vi "GetDisabledInputs.vi"(6 "error in":errorcluster, 9 "IndexArray in":refnum<class "IndexArray.lvclass">) -> (0 "error out":errorcluster, 3 "IndexArray out":refnum<class "IndexArray.lvclass">, 4 "indices":string)   [LabVIEW 2014, in "IndexArray.lvclass"]
uses:
  IndexArray.lvclass
  Python/Parsing/ListTypesTD.ctl
  Python/Parsing/Python Functions.lvlib
  Python/PythonConfiguration/PythonConfiguration.lvclass
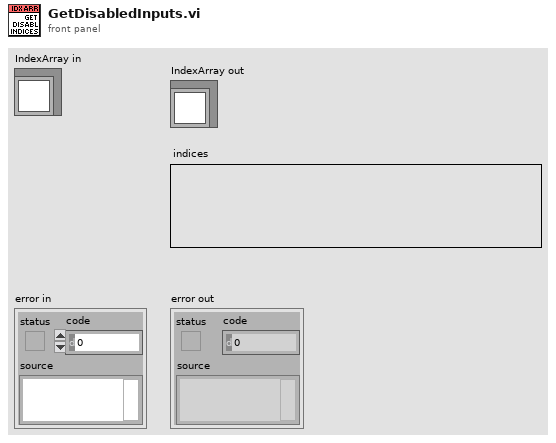
[diagram p1: front panel]
types:
  T1 = typedef "Python Functions.lvlib/ListTypesTD.ctl" = enum16{"list", "tuple", "parameter list", "output list", "return values"}
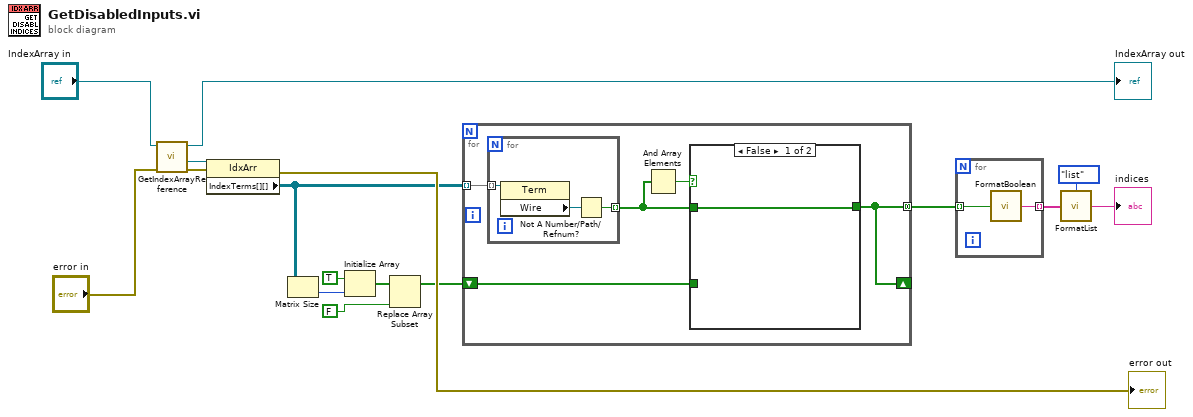
[diagram p0: block diagram]
diagram:
  n1 = call "GetIndexArrayReference.vi"("error in"="error in", "Index Array in"="IndexArray in") -> ("error out"=w13:errorcluster, "reference out"=w14:refnum<vi>, "Index Array out"=→"IndexArray out":refnum<class "IndexArray.lvclass">)  [unwired: 7 in]
  n2 = property class="IdxArr"(reference=w14, error in=w13) -> (error out=→"error out":errorcluster, "IndexTerms[][]"=w2:refnum<vi>[][])  [unwired: 1 out]
  n3 = Matrix Size(0:w2) -> (2:w1:i32)  [unwired: 1 out]
  n4 = Initialize Array(TRUE, w1) -> (w6:bool[])
  n5 = Replace Array Subset(array=w6, new element=FALSE) -> (w4:bool[])  [unwired: 1 in]
  n6 = for {
    tunnel: w2 -> [w21] mode=indexing
    shift-right: [w17] -> _
    shift-left: w4 -> [w18]
    tunnel: [w17] -> w3 mode=concatenating
    n7 = for {
      tunnel: w21 -> [w26] mode=indexing
      tunnel: [w25] -> w20 mode=indexing
      n8 = property class="Term"(reference=w26) -> ("Wire"=w24:refnum<vi>)  [unwired: 1 in, 2 out]
      n9 = Not A Number/Path/Refnum?(number/path/refnum=w24) -> (NaN/Path/Refnum?=w25:bool)
    }
    n10 = And Array Elements(Boolean array=w20) -> (logical AND=w19:bool)
    n11 = case shown="False" w19 {
      tunnel: w20 -> [w22 _]
      tunnel: w18 -> [_ w23]
      tunnel: [w22 w23] -> w17
      frame False {
      }
      frame True {
      }
    }
  }
  n12 = for {
    tunnel: w3 -> [w28] mode=indexing
    tunnel: [w27] -> w9 mode=indexing
    n13 = call "FormatBoolean.vi"("boolean"=w28) -> ("value"=w27:string)
  }
  n14 = call "FormatList.vi"("values"=w9, "type"=ListTypesTD."list") -> ("python object"=→"indices":string)
